vi "Kalman filter - P array 2nd (SubVI).vi"(1 "P Array in":dbl[][](array[numeric]), 2 "K Array in":dbl[](array[numeric])) -> (0 "P Array out":dbl[][](array[numeric]))   [LabVIEW 2013]
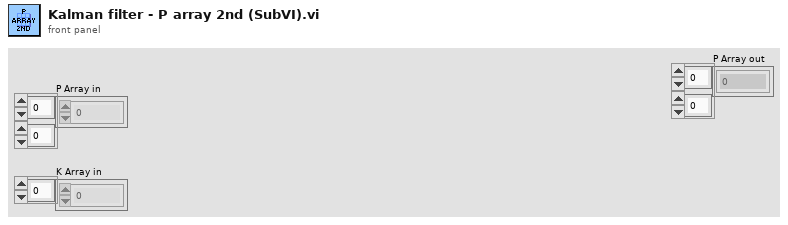
[diagram p1: front panel]
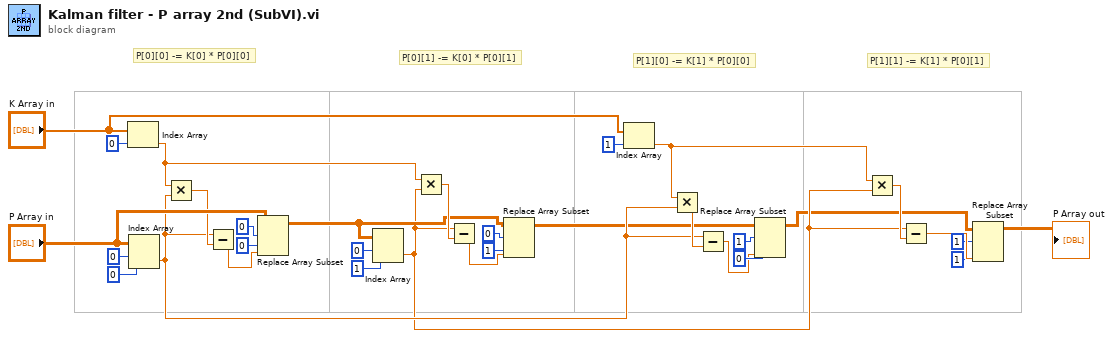
[diagram p0: block diagram]
diagram:
  # "P[1][1] -= K[1] * P[0][1]"
  # "P[1][0] -= K[1] * P[0][0]"
  # "P[0][1] -= K[0] * P[0][1]"
  # "P[0][0] -= K[0] * P[0][0]"
  n1 = Index Array(array="K Array in", index=0) -> (element=w22:dbl)
  n2 = Index Array(array="P Array in", index (row)=0, index (col)=0 ("disabled index (col)")) -> (element=w11:dbl)
  n3 = Multiply(x=w22, y=w11) -> (x*y=w28:dbl)
  n4 = Subtract(x=w11, y=w28) -> (x-y=w32:dbl)
  n5 = Replace Array Subset(array="P Array in", new element=w32, index (row)=0, index (col)=0 ("disabled index (col)")) -> (w18:dbl[][])
  n6 = Index Array(array=w18, index (row)=0, index (col)=1 ("disabled index (col)")) -> (element=w6:dbl)
  n7 = Multiply(x=w22, y=w6) -> (x*y=w21:dbl)
  n8 = Subtract(x=w6, y=w21) -> (x-y=w17:dbl)
  n9 = Replace Array Subset(array=w18, new element=w17, index (row)=0, index (col)=1) -> (w9:dbl[][])
  n10 = Index Array(array="K Array in", index=1) -> (element=w8:dbl)
  n11 = Multiply(x=w8, y=w11) -> (x*y=w12:dbl)
  n12 = Subtract(x=w11, y=w12) -> (x-y=w10:dbl)
  n13 = Replace Array Subset(array=w9, new element=w10, index (row)=1, index (col)=0) -> (w2:dbl[][])
  n14 = Multiply(x=w8, y=w6) -> (x*y=w7:dbl)
  n15 = Subtract(x=w6, y=w7) -> (x-y=w5:dbl)
  n16 = Replace Array Subset(array=w2, new element=w5, index (row)=1, index (col)=1) -> (→"P Array out":dbl[][])
